vi "Point Equal.vi"(1 "Point B":cluster{"X":dbl, "Y":dbl}, 2 "Point A":cluster{"X":dbl, "Y":dbl}) -> (0 "Equal":bool)   [LabVIEW 2017]
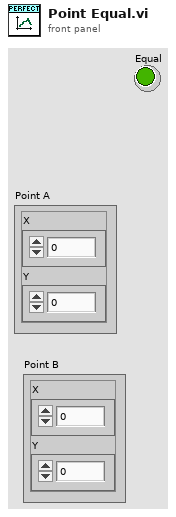
[diagram p1: front panel]
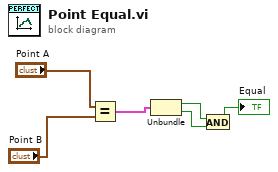
[diagram p0: block diagram]
diagram:
  n1 = Equal?(x="Point A", y="Point B") -> (x = y?=w4:cluster{"X":bool, "Y":bool})
  n2 = Unbundle(w4) -> ("X"=w3:bool, "Y"=w2:bool)
  n3 = And(x=w3, y=w2) -> (x .and. y?=→"Equal":bool)
